vi "SW_Determine_path_to_Load.vi"(10 "Load Settings from File Argument":T1, 11 "App.Kind":T2(ring)) -> (1 "Researcher name":string, 2 "User Settings path":path, 3 "Program Settings path":path)   [LabVIEW 2018, in "Settings.lvlib"]
uses:
  Settings.lvlib
  Load Settings from File Argument--cluster.ctl
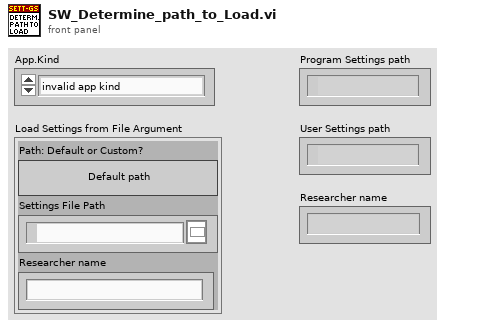
[diagram p1: front panel]
types:
  T1 = typedef "Settings.lvlib/Load Settings from File Argument--cluster.ctl" = cluster{"Path: Default or Custom?":bool, "Settings File Path":path, "Researcher name":string}
  T2 = enum32{"invalid app kind", "Development System", "Run Time System", "Student Edition", "Embedded LabVIEW", "Evaluation", "Custom"}
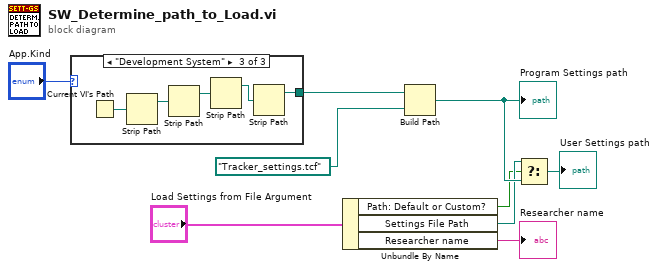
[diagram p0: block diagram]
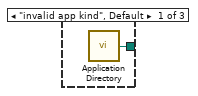
[diagram p2: hidden frame]
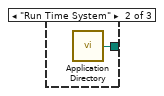
[diagram p3: hidden frame]
diagram:
  n1 = case shown="\"Development System\"" "App.Kind" {
    tunnel: [w10 w11 w12] -> w2
    frame "invalid app kind", Default {
      n2 = call <vilib>:"Application Directory.vi"() -> ("Application Directory"=w10:path)
    }
    frame "Run Time System" {
      n3 = call <vilib>:"Application Directory.vi"() -> ("Application Directory"=w11:path)
    }
    frame "Development System" {
      n4 = Current VI's Path() -> (path=w16:path)
      n5 = Strip Path(path=w16) -> (stripped path=w15:path)  [unwired: 1 out]
      n6 = Strip Path(path=w15) -> (stripped path=w14:path)  [unwired: 1 out]
      n7 = Strip Path(path=w14) -> (stripped path=w13:path)  [unwired: 1 out]
      n8 = Strip Path(path=w13) -> (stripped path=w12:path)  [unwired: 1 out]
    }
  }
  n9 = Unbundle By Name("Load Settings from File Argument") -> ("Path: Default or Custom?"=w4:bool, "Settings File Path"=w6:path, "Researcher name"=→"Researcher name":string)
  n10 = Build Path(base path=w2, name or relative path=path "Tracker_settings.tcf") -> (appended path=w9:path)
  "Program Settings path" <- w9
  n11 = Select(t=w6, s=w4, f=w9) -> (s? t:f=→"User Settings path":path)
